vi "Start CAN.vi"(8 "错误输入（无错误）":errorcluster caption="Error In(No Error)", 11 "CAN Device In":T1={"Device Type"=20, "Device Index"=0, "CANInd"=0, "Baud(E_U)"=1835016} {"Baud(E_U)" items=["1000Kbps"=393219, "800Kbps"=393220, "500Kbps"=393223, "250Kbps"=1835016, "125Kbps"=1835025, "100Kbps"=1441827, "50Kbps"=1835052, "20Kbps"=1441971, "10Kbps"=1835232, "5Kbps"=1835457]; "Device Type" items=["PCI5121"=1, "PCI9810"=2, "USBCAN1"=3, "USBCAN2"=4, "PCI9820"=5, "PCI5110"=7, "PC104CAN"=11, "CANETUDP"=12, "PCI9840B"=14, "PC104C2"=15, "PCI9820I"=16, "CANETTCP"=17, "PCIE9221"=24, "PCI5010U"=19, "USBCAN_E_U"=20, "USBCAN_2E_U"=21, "PCI5020U"=22, "PCIE9120I"=27, "PCIE9110I"=28, "PCIE9140I"=29, "USBCAN-4E-U"=31, "USBCAN-8E-U"=34]}) -> (0 "错误输出":errorcluster caption="Error Out", 1 "Start成功？":bool, 3 "CAN Device Out":T1={"Device Type"=20, "Device Index"=0, "CANInd"=0, "Baud(E_U)"=1835016} {"Baud(E_U)" items=["1000Kbps"=393219, "800Kbps"=393220, "500Kbps"=393223, "250Kbps"=1835016, "125Kbps"=1835025, "100Kbps"=1441827, "50Kbps"=1835052, "20Kbps"=1441971, "10Kbps"=1835232, "5Kbps"=1835457]; "Device Type" items=["PCI5121"=1, "PCI9810"=2, "USBCAN1"=3, "USBCAN2"=4, "PCI9820"=5, "PCI5110"=7, "PC104CAN"=11, "CANETUDP"=12, "PCI9840B"=14, "PC104C2"=15, "PCI9820I"=16, "CANETTCP"=17, "PCIE9221"=24, "PCI5010U"=19, "USBCAN_E_U"=20, "USBCAN_2E_U"=21, "PCI5020U"=22, "PCIE9120I"=27, "PCIE9110I"=28, "PCIE9140I"=29, "USBCAN-4E-U"=31, "USBCAN-8E-U"=34]})   [LabVIEW 2020, in "ZLGCAN.lvclass"]
uses:
  ZLGCAN.lvclass
  Device.ctl
  <vilib>/ErrorRing/Error Ring.xnode
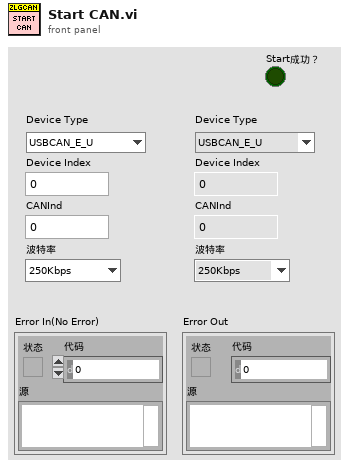
[diagram p1: front panel]
types:
  T1 = typedef "ZLGCAN.lvclass/Device.ctl" = cluster{"Device Type":u32, "Device Index":u32, "CANInd":u32, "Baud(E_U)":u32}
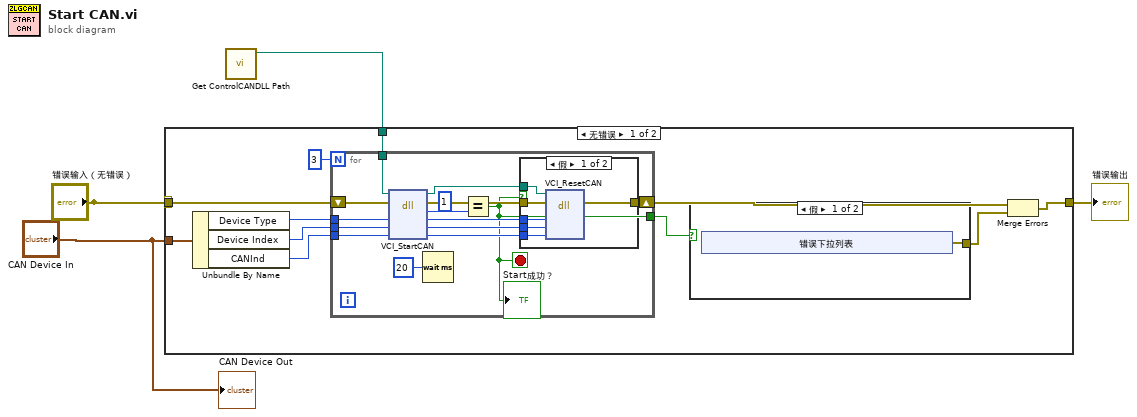
[diagram p0: block diagram]
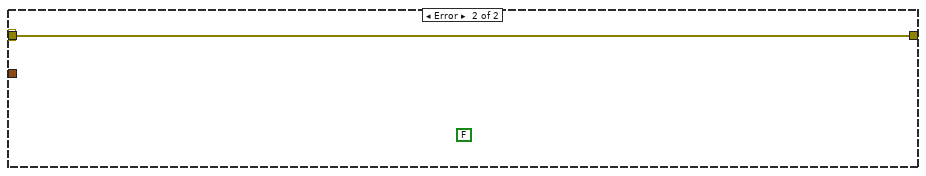
[diagram p4: hidden frame]
diagram:
  n1 = call "Get ControlCANDLL Path.vi"() -> ("拆分的路径"=w1:path)  [unwired: 10 in, 1 out]
  n2 = case shown="无错误" "错误输入（无错误）" {
    tunnel: "错误输入（无错误）" -> [w12 w40]
    tunnel: [w13 w40] -> w3
    tunnel: "CAN Device In" -> [w10 _]
    tunnel: w1 -> [w5 _]
    frame No Error {
      n3 = Unbundle By Name(w10) -> ("Device Type"=w7:u32, "Device Index"=w8:u32, "CANInd"=w9:u32)
      n4 = for {
        N: 3 -> [_]
        tunnel: [w18] -> w14
        tunnel: w9 -> [w29]
        tunnel: w8 -> [w28]
        tunnel: w7 -> [w27]
        shift-right: [w19] -> w11
        shift-left: w12 -> [w30]
        tunnel: w5 -> [w17]
        stop <- w18 stop-if-true
        n5 = dll-call lib="D:/eDMT Monitor/support/ZLG CAN/ControlCAN.dll" fn="VCI_StartCAN"(path in=w17, error in=w30, "DeviceType"=w27, "DeviceInd"=w28, "CANInd"=w29) -> (path out=w16:path, error out=w25:errorcluster, "返回类型"=w22:u32, "DeviceType"=w24:u32, "DeviceInd"=w21:u32, "CANInd"=w20:u32)  [unwired: 1 in]
        n6 = Wait (ms)(milliseconds to wait=u32 20 ("等待时间（毫秒）")) -> ()  [unwired: 1 out]
        n7 = Equal?(x=u32 1 ("y"), y=w22) -> (x = y?=w18:bool)
        "Start成功？" <- w18
        n8 = case shown="假" w18 {
          tunnel: w25 -> [w36 w37]
          tunnel: w24 -> [w35 _]
          tunnel: w21 -> [w34 _]
          tunnel: w20 -> [w33 _]
          tunnel: [w32 w37] -> w19
          tunnel: w16 -> [w31 _]
          frame False {
            n9 = dll-call lib="D:/eDMT Monitor/support/ZLG CAN/ControlCAN.dll" fn="VCI_ResetCAN"(path in=w31, error in=w36, "DeviceType"=w35, "DeviceInd"=w34, "CANInd"=w33) -> (error out=w32:errorcluster)  [unwired: 4 in, 2 out]
          }
          frame True {
          }
        }
      }
      n10 = case shown="假" w14 {
        tunnel: [w38 _] -> w15
        frame False {
          n11 = xnode "错误下拉列表"() -> ("错误输出"=w38:errorcluster)
        }
        frame True {
        }
      }
      n12 = Merge Errors(w11, w15) -> (w13:errorcluster)
    }
    frame Error {
      (unwired) FALSE
    }
  }
  "错误输出" <- w3
  "CAN Device Out" <- "CAN Device In"
